vi "Interface.vi"() -> ()   [LabVIEW 2023]
panel:
  in  "Arduino Load Cell Readings?":refnum<visa-resource-name>
  in  "Frequency":dbl
  in  "VISA resource name":refnum<visa-resource-name>
  in  "number of times to repeat":string caption="n"
  in  "desired strain %":dbl
  in  "sample length (mm)":dbl
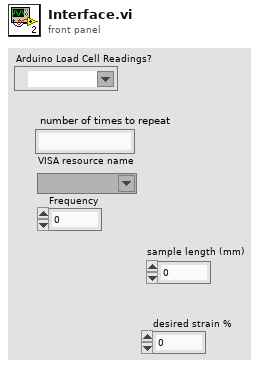
[diagram p1: front panel]
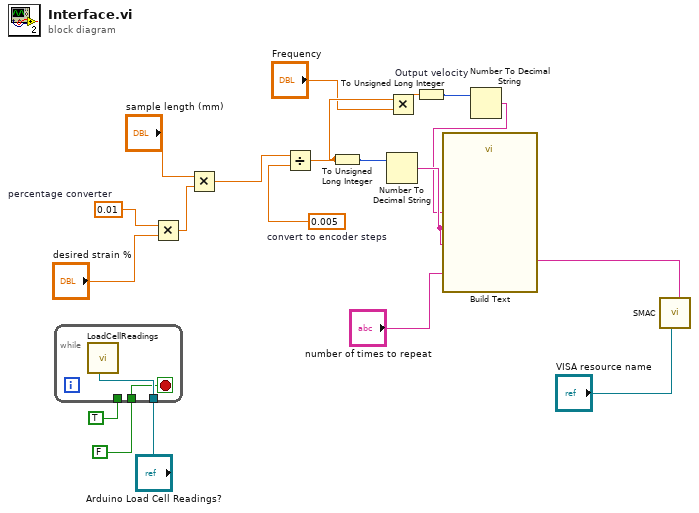
[diagram p0: block diagram]
diagram:
  w14 = 0.005  # convert to encoder steps
  w17 = 0.01  # percentage converter
  n1 = while {
    tunnel: TRUE -> [_]
    tunnel: "Arduino Load Cell Readings?" -> [w21]
    tunnel: FALSE -> [w20]
    stop <- w20 stop-if-true
    n2 = call "LoadCellReadings.vi"("Arduino Load Cell Readings?"=w21) -> ()  [unwired: 11 in]
  }
  n3 = Multiply(x=w17, y="desired strain %") -> (x*y=w16:dbl)
  n4 = Multiply(x="sample length (mm)", y=w16) -> (x*y=w15:dbl)
  n5 = Divide(x=w15, y=w14) -> (x/y=w6:dbl)
  n6 = To Unsigned Long Integer(number=w6) -> (unsigned 32bit integer=w11:u32)
  n7 = Number To Decimal String(number=w11) -> (decimal integer string=w8:string)  [unwired: 1 in]
  n8 = Multiply(x=w6, y="Frequency") -> (x*y=w4:dbl)
  n9 = To Unsigned Long Integer "Output velocity"(number=w4) -> (unsigned 32bit integer=w10:u32)
  n10 = Number To Decimal String(number=w10) -> (decimal integer string=w7:string)  [unwired: 1 in]
  n11 = call "Build Text"("n"="number of times to repeat", "vel"=w7, "counts"=w8, "counts2"=w8) -> ("Result"=w12:string)  [unwired: 10 in, 1 out]
  n12 = call "SMAC.vi"("write buffer"=w12, "VISA resource name"="VISA resource name") -> ()  [unwired: 10 in]
